vi "close.vi"(5 ".NET Refnum in":refnum<k24>, 6 "DigitizerIdVarPtr":refnum<k24>, 7 "ContextAppVarPtr":refnum<k24>, 8 "error in (no error)":errorcluster, 9 "DisplayIdVarPtr":refnum<k24>, 10 "SystemIdVarPtr":refnum<k24>, 11 ".NET Refnum in":refnum<k24>) -> (0 "error out":errorcluster)   [LabVIEW 2019]
uses:
  C:/Users/huang/Desktop/MIL LITE 10/64/Matrox Imaging/MIL/MIL.NET/Matrox.MatroxImagingLibrary.v3.5.dll
  64/Matrox Imaging/MIL/MIL.NET/Matrox.MatroxImagingLibrary.v3.5.dll
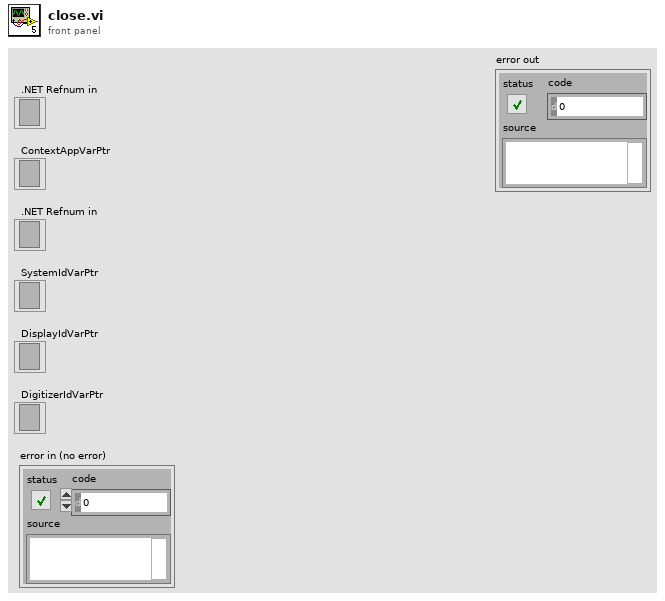
[diagram p1: front panel]
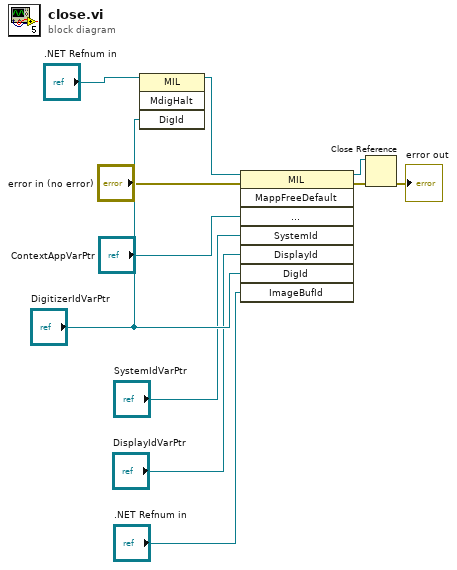
[diagram p0: block diagram]
diagram:
  n1 = invoke on="调用节点" class="MIL" method="MdigHalt"(reference=".NET Refnum in", "DigId"="DigitizerIdVarPtr") -> (reference out=w9:refnum<k24>)  [unwired: 2 in, 3 out]
  n2 = invoke on="调用节点" class="MIL" method="MappFreeDefault"(reference=w9, error in="error in (no error)", "ApplicationId"="ContextAppVarPtr", "SystemId"="SystemIdVarPtr", "DisplayId"="DisplayIdVarPtr", "DigId"="DigitizerIdVarPtr", "ImageBufId"=".NET Refnum in") -> (reference out=w3:refnum<k24>, error out=w5:errorcluster)  [unwired: 1 in, 6 out]
  n3 = Close Reference(reference=w3, error in (no error)=w5) -> (error out=→"error out":errorcluster)
